vi "Actor Core.vi"(8 "error in":errorcluster, 11 "Nested in":refnum<class "Text based Communications Test.lvclass">) -> (0 "error out":errorcluster, 3 "Actor out":refnum<class "Actor.lvclass">)   [LabVIEW 2017, in "Text based Communications Test.lvlib" / "Text based Communications Test.lvclass"]
doc: "(<B>Filename</B>: Actor Framework.lvlib:Actor.lvclass:Actor Core.vi)\n\nReceives messages to the actor, reacts to them, and initiates any error handling that may shut the actor down.\n\nDescendant classes may override this VI to append parallel tasks for the actor to complete while it handles messages. Overrides use the Call Parent Method node."
uses:
  Text based Communications Test.lvclass
  C:/Program Files (x86)/National Instruments/LabVIEW 2017/vi.lib/ActorFramework/Actor/Actor.lvclass
  <vilib>/ActorFramework/Actor/Actor.lvclass
  File based Comm Helper Loop States.ctl
  <vilib>/ActorFramework/Message Enqueuer/Message Enqueuer.lvclass
  File Data Format.ctl
  Text based Communications Test.lvclass/Text based Communications Test.ctl
  <vilib>/ActorFramework/Actor/Actor.lvclass/Actor.ctl
  <vilib>/ActorFramework/Message Enqueuer/Message Enqueuer.lvclass/Message Enqueuer.ctl
  Test/Test Messages/Update Test Progress Msg/Update Test Progress Msg.lvclass/Update Test Progress Msg.ctl
  Text based Communications Test Messages/Validate Response Msg/Validate Response Msg.lvclass/Validate Response Msg.ctl
  <vilib>/ActorFramework/Message Enqueuer/Init from Existing Queue.vi
  <vilib>/ActorFramework/Message Enqueuer/Enqueue.vi
  Test/Test Messages/Update Test Progress Msg/Update Test Progress Msg.lvclass
  C:/Program Files (x86)/National Instruments/LabVIEW 2017/vi.lib/ActorFramework/Message/Message.lvclass
  Text based Communications Test Messages/Validate Response Msg/Validate Response Msg.lvclass
  <vilib>/ActorFramework/Message Priority Queue/Priority Enqueue.vi
  Test/Test/Test.lvclass
  Text based Communications Test.lvlib
panel:
  out "Table":i32[](listbox)
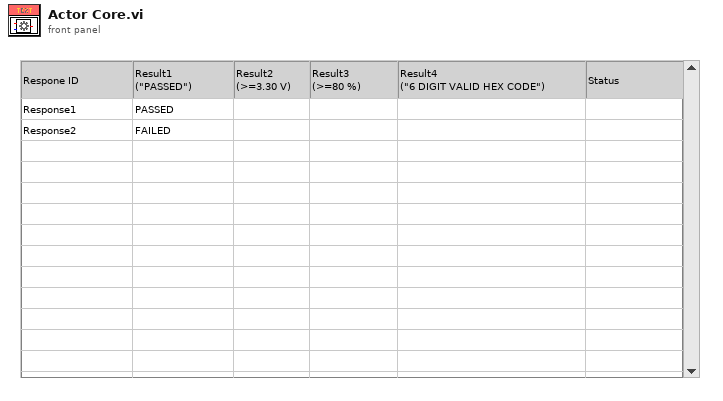
[diagram p1: front panel]
types:
  T1 = typedef "Text based Communications Test.lvlib/File Data Format.ctl" = cluster{"Response ID":string, "Value":cluster{"Result1":string, "Result2":dbl, "Result3":string, "Result4":string}}
  T2 = cluster{"Self Enqueuer":refnum<class "Message Enqueuer.lvclass">, "raw text":string, "File Type":string, "Array":T1[], "Test Name":string, "Test Configuration":cluster{"Path":path}}
  T3 = typedef "Text based Communications Test.lvlib/File based Comm Helper Loop States.ctl" = enum16{"Poll", "Init", "Read Test Case", "Read Input Text File", "Parse Data", "Validate", "Update Result", "Stream Data to Actor", "Error", "Exit"}
  T4 = typedef "Paths.ctl" = cluster{"Data Directory":path, "Test Config Dir":path, "Error Logs":path, "Event Logs":path, "Settings.Json":path, "Reports Directory":path}
  T5 = cluster{"Response ID":string, "Value":cluster{"Result1":string, "Result2":dbl, "Result3":string, "Result4":string}}[]
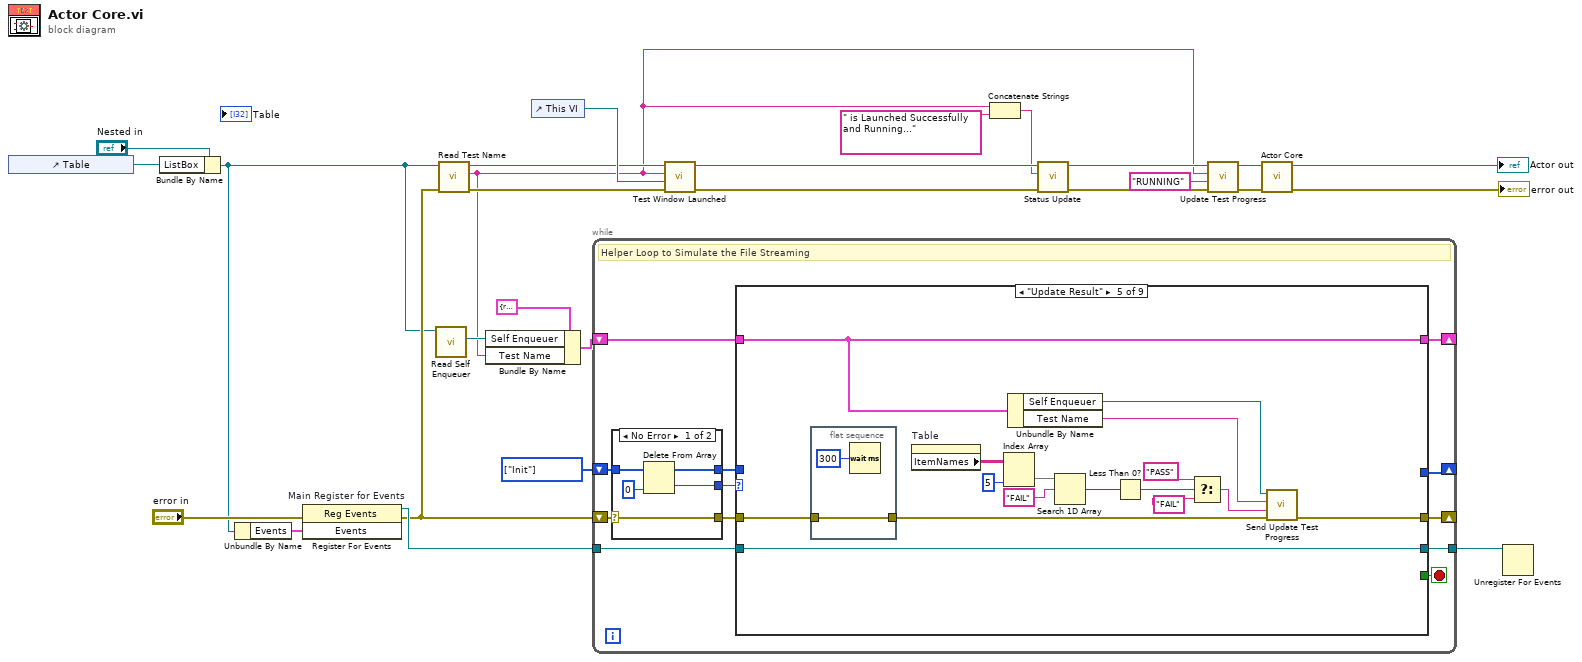
[diagram p0: block diagram]
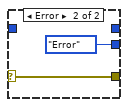
[diagram p2: hidden frame]
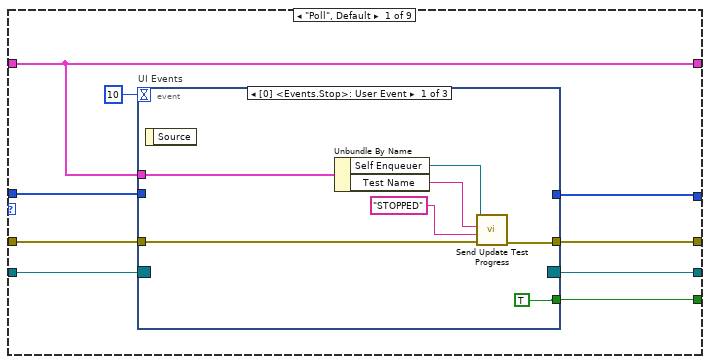
[diagram p3: hidden frame]
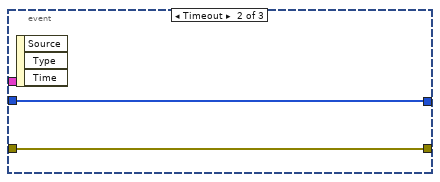
[diagram p4: hidden frame]
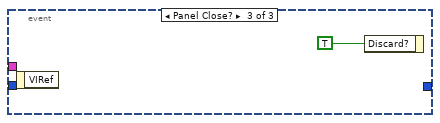
[diagram p5: hidden frame]
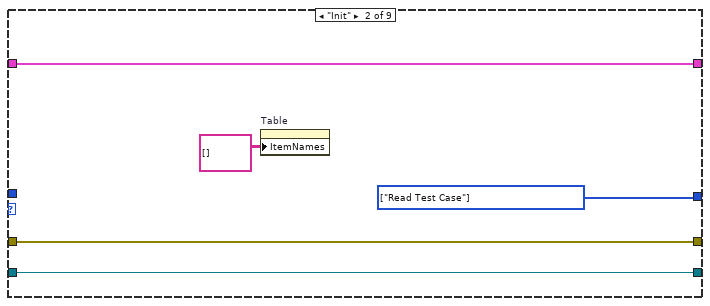
[diagram p6: hidden frame]
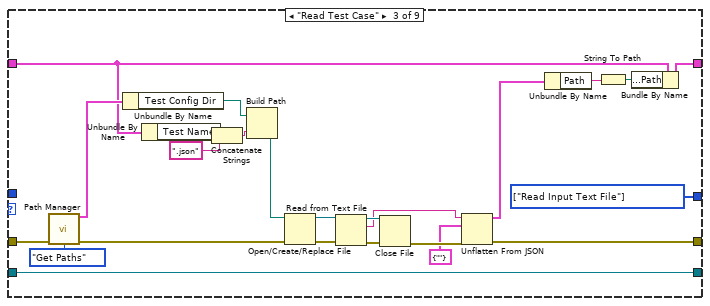
[diagram p7: hidden frame]
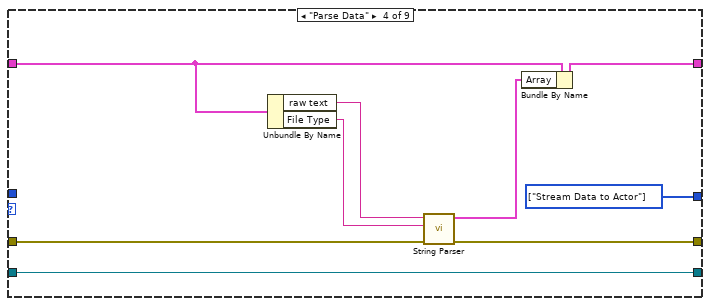
[diagram p8: hidden frame]
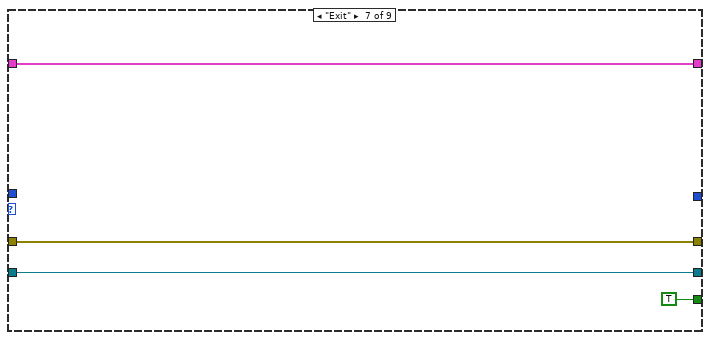
[diagram p10: hidden frame]
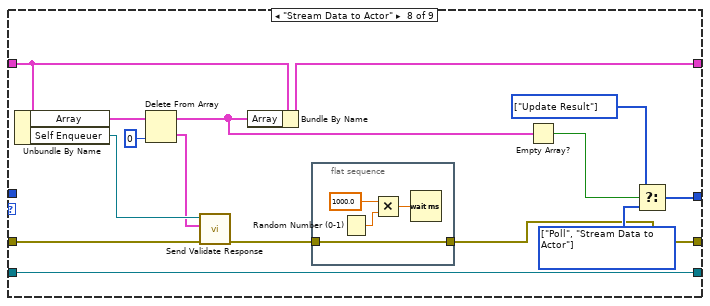
[diagram p11: hidden frame]
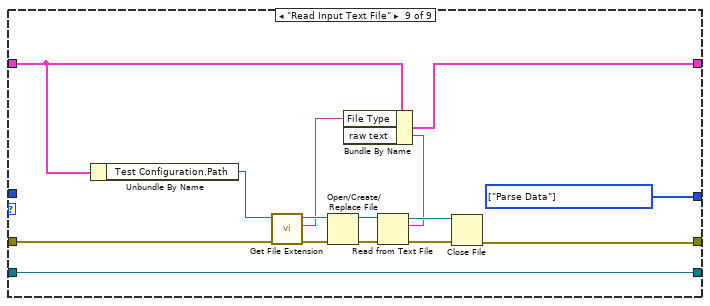
[diagram p12: hidden frame]
diagram:
  w17 = T3[] [enum."Init"] items=["Poll", "Init", "Read Test Case", "Read Input Text File", "Parse Data", "Validate", "Update Result", "Stream Data to Actor", "Error", "Exit"]
  n1 = control-ref of="Table"() -> (w2:refnum<vi>)
  n2 = Bundle By Name(cluster="Nested in", "ListBox"=w2) -> (w3:refnum<class "Text based Communications Test.lvclass">)
  n3 = Unbundle By Name(w3) -> ("Events"=w22:cluster{"Stop":refnum<user-event>})
  n4 = register-events "Main Register for Events"(error in="error in", w22) -> (reference out=w23:refnum<event-registration>, error out=w18:errorcluster)  [unwired: 1 in]
  n5 = call <vilib>:"Read Self Enqueuer.vi"("Actor"=w3) -> ("Self Enqueuer"=w4:refnum<class "Message Enqueuer.lvclass">)  [unwired: 10 in]
  n6 = call-dynamic "Read Test Name.vi"("Test in"=w3) -> ("Test Name"=w1:string, "Test out"=w10:refnum<class "Text based Communications Test.lvclass">)  [unwired: 8 in, 1 out]
  n7 = Bundle By Name(cluster=T2 {"Self Enqueuer"=refnum, "raw text"="", "File Type"="", "Array"=[], "Test Name"="", "Test Configuration"={"Path"=path ""}}, "Self Enqueuer"=w4, "Test Name"=w1) -> (w5:T2)
  n8 = control-ref of="This VI"() -> (w19:refnum<vi>)
  n9 = while {
    tunnel: w23 -> [w37]
    tunnel: [w35] -> w21
    shift-right: [w30] -> _
    shift-left: w17 -> [w31]
    shift-right: [w34] -> _
    shift-left: w18 -> [w32]
    shift-right: [w28] -> _
    shift-left: w5 -> [w29]
    stop <- w36 stop-if-true
    # "Helper Loop to Simulate the File Streaming"
    n10 = case shown="No Error" w32 {
      selector: w32 -> [w41 w44]
      tunnel: [w41 w44] -> w33
      tunnel: w31 -> [w42 _]
      tunnel: [w40 _] -> w26
      tunnel: [w38 File_based_Comm_Helper_Loop_States."Error" ("Enum")] -> w27
      frame No Error {
        n11 = Delete From Array(array=w42, index=0) -> (deleted portion=w38:T3, array with subset deleted=w40:T3[])  [unwired: 1 in]
      }
      frame Error {
      }
    }
    n12 = case shown="\"Update Result\"" w27 {
      tunnel: w37 -> [w53 w68 w92 w101 w117 w122 w124 w141 w160]
      tunnel: [w52 _ _ _ _ _ TRUE _ _] -> w36
      tunnel: [w51 w68 w92 w101 w117 w122 w124 w141 w160] -> w35
      tunnel: w33 -> [w50 w67 w91 w100 w103 w120 w126 w130 w154]
      tunnel: [w48 w67 w76 w99 w104 w120 w126 w127 w150] -> w34
      tunnel: [w46 w64 w69 w93 _ _ _ w133 w149] -> w30
      tunnel: w29 -> [w45 w66 w74 w96 w105 w121 w123 w140 w147]
      tunnel: [w45 w66 w73 w98 w105 w121 w123 w137 w148] -> w28
      tunnel: w26 -> [w47 _ _ _ _ _ _ _ _]
      frame "Poll", Default {
        n13 = event "UI Events" shown="[0] <Events.Stop>: User Event" {
          selector: w53 -> [_ _ _]
          dyn-events: [_ _ _] -> w51
          timeout: 10 -> [_ _ _]
          tunnel: [TRUE _ _] -> w52
          tunnel: w50 -> [w55 w62 _]
          tunnel: [w54 w62 _] -> w48
          tunnel: w47 -> [_ w61 _]
          tunnel: [_ w61 _] -> w46
          tunnel: w45 -> [w57 _ _]
          event User Event {
            n14 = event-data() -> ()  [unwired: 1 in, 1 out]
            n15 = Unbundle By Name(w57) -> ("Self Enqueuer"=w56:refnum<class "Message Enqueuer.lvclass">, "Test Name"=w58:string)
            n16 = call "Send Update Test Progress.vi"("error in (no error)"=w55, "State"="STOPPED", "Test Name"=w58, "Message Enqueuer"=w56) -> ("error out"=w54:errorcluster)  [unwired: 6 in, 1 out]
          }
          event Timeout {
            n17 = event-data() -> ()  [unwired: 1 in, 3 out]
          }
          event Panel Close? {
            n18 = event-data() -> ()  [unwired: 1 in, 1 out]
            n19 = event-data("Discard?"=TRUE) -> ()  [unwired: 1 in, 1 out]
          }
        }
      }
      frame "Init" {
        w64 = T3[] [enum."Read Test Case"] items=["Poll", "Init", "Read Test Case", "Read Input Text File", "Parse Data", "Validate", "Update Result", "Stream Data to Actor", "Error", "Exit"] ("t")
        n20 = property on="Table" class="MCListbox (strict)"("ItemNames"=string[][] [] ("Item Names")) -> ()  [unwired: 2 in, 2 out]
      }
      frame "Read Test Case" {
        w69 = T3[] [enum."Read Input Text File"] items=["Poll", "Init", "Read Test Case", "Read Input Text File", "Parse Data", "Validate", "Update Result", "Stream Data to Actor", "Error", "Exit"] ("t")
        n21 = call "Path Manager.vi"("Error in (no error)"=w91, "Options"=enum16{"Get Paths", "Init Paths"}."Get Paths") -> ("Cluster"=w89:T4, "Error out"=w80:errorcluster)  [unwired: 12 in]
        n22 = Unbundle By Name(w89) -> ("Test Config Dir"=w88:path)
        n23 = Unbundle By Name(w74) -> ("Test Name"=w87:string)
        n24 = Concatenate Strings(w87, ".json" ("string")) -> (w86:string)
        n25 = Build Path(base path=w88, name or relative path=w86) -> (appended path=w79:path)
        n26 = Open/Create/Replace File(file path (use dialog)=w79, error in=w80) -> (refnum out=w83:refnum<file>, error out=w84:errorcluster)  [unwired: 4 in, 1 out]
        n27 = Read from Text File(file (use dialog)=w83, error in=w84) -> (refnum out=w81:refnum<file>, text=w78:string, error out=w82:errorcluster)  [unwired: 2 in, 1 out]
        n28 = Close File(refnum=w81, error in=w82) -> (error out=w77:errorcluster)  [unwired: 1 out]
        n29 = Unflatten From JSON(JSON string=w78, type and defaults=cluster{"Path":string} {"Path"=""}, error in (no error)=w77) -> (value=w72:cluster{"Path":string}, error out=w76:errorcluster)  [unwired: 4 in]
        n30 = Unbundle By Name(w72) -> ("Path"=w71:string)
        n31 = String To Path(string=w71) -> (path=w70:path)
        n32 = Bundle By Name(cluster=w74, "Test Configuration.Path"=w70) -> (w73:T2)
      }
      frame "Parse Data" {
        w93 = T3[] [enum."Stream Data to Actor"] items=["Poll", "Init", "Read Test Case", "Read Input Text File", "Parse Data", "Validate", "Update Result", "Stream Data to Actor", "Error", "Exit"]
        n33 = Unbundle By Name(w96) -> ("raw text"=w95:string, "File Type"=w94:string)
        n34 = call "String Parser.vi"("Error in (no error)"=w100, "File Type"=w94, "raw string"=w95) -> ("Error out"=w99:errorcluster, "Array"=w97:T5)  [unwired: 7 in]
        n35 = Bundle By Name(cluster=w96, "Array"=w97) -> (w98:T2)
      }
      frame "Update Result" {
        n36 = flat-sequence {
          tunnel: w103 -> [w119]
          tunnel: [w119] -> w102
          frame #0 {
            n37 = Wait (ms)(milliseconds to wait=u32 300) -> ()  [unwired: 1 out]
          }
        }
        n38 = property on="Table" class="MCListbox (strict)"() -> ("ItemNames"=w106:string[][])  [unwired: 2 in, 2 out]
        n39 = Index Array(array=w106, index (col)=5 ("disabled index (col)")) -> (element=w113:string[])  [unwired: 1 in]
        n40 = Unbundle By Name(w105) -> ("Self Enqueuer"=w116:refnum<class "Message Enqueuer.lvclass">, "Test Name"=w115:string)
        n41 = Search 1D Array(1D array=w113, element="FAIL") -> (index of element=w111:i32)  [unwired: 1 in]
        n42 = Less Than 0?(x=w111) -> (x < 0?=w110:bool)
        n43 = Select(t="PASS" ("State"), s=w110, f="FAIL" ("State")) -> (s? t:f=w107:string)
        n44 = call "Send Update Test Progress.vi"("error in (no error)"=w102, "State"=w107, "Test Name"=w115, "Message Enqueuer"=w116) -> ("error out"=w104:errorcluster)  [unwired: 6 in, 1 out]
      }
      frame "Error" {
      }
      frame "Exit" {
      }
      frame "Stream Data to Actor" {
        w129 = T3[] [enum."Update Result"] items=["Poll", "Init", "Read Test Case", "Read Input Text File", "Parse Data", "Validate", "Update Result", "Stream Data to Actor", "Error", "Exit"] ("t")
        w134 = T3[] [enum."Poll", enum."Stream Data to Actor"] items=["Poll", "Init", "Read Test Case", "Read Input Text File", "Parse Data", "Validate", "Update Result", "Stream Data to Actor", "Error", "Exit"]
        n45 = Unbundle By Name(w140) -> ("Array"=w139:T1[], "Self Enqueuer"=w132:refnum<class "Message Enqueuer.lvclass">)
        n46 = Delete From Array(array=w139, index=0) -> (deleted portion=w131:T1, array with subset deleted=w136:T1[])  [unwired: 1 in]
        n47 = call "Send Validate Response.vi"("error in (no error)"=w130, "Response Data"=w131, "Message Enqueuer"=w132) -> ("error out"=w128:errorcluster)  [unwired: 7 in, 1 out]
        n48 = Bundle By Name(cluster=w140, "Array"=w136) -> (w137:T2)
        n49 = flat-sequence {
          tunnel: w128 -> [w145]
          tunnel: [w145] -> w127
          frame #0 {
            n50 = Random Number (0-1)() -> (number: 0 to 1=w144:dbl)
            n51 = Multiply(x=1000.0, y=w144) -> (x*y=w142:dbl)
            n52 = Wait (ms)(milliseconds to wait=w142) -> ()  [unwired: 1 out]
          }
        }
        n53 = Empty Array?(array=w136) -> (empty?=w135:bool)
        n54 = Select(t=w129, s=w135, f=w134) -> (s? t:f=w133:T3[])
      }
      frame "Read Input Text File" {
        w149 = T3[] [enum."Parse Data"] items=["Poll", "Init", "Read Test Case", "Read Input Text File", "Parse Data", "Validate", "Update Result", "Stream Data to Actor", "Error", "Exit"]
        n55 = Unbundle By Name(w147) -> ("Test Configuration.Path"=w146:path)
        n56 = call <vilib>:"Get File Extension.vi"("error in (no error)"=w154, "file"=w146) -> ("error out"=w153:errorcluster, "lowercase file extension"=w155:string, "dup file"=w156:path)  [unwired: 5 in, 2 out]
        n57 = Open/Create/Replace File(file path (use dialog)=w156, error in=w153) -> (refnum out=w159:refnum<file>, error out=w152:errorcluster)  [unwired: 4 in, 1 out]
        n58 = Read from Text File(file (use dialog)=w159, error in=w152) -> (refnum out=w158:refnum<file>, text=w157:string, error out=w151:errorcluster)  [unwired: 2 in, 1 out]
        n59 = Bundle By Name(cluster=w147, "File Type"=w155, "raw text"=w157) -> (w148:T2)
        n60 = Close File(refnum=w158, error in=w151) -> (error out=w150:errorcluster)  [unwired: 1 out]
      }
    }
  }
  n61 = call-dynamic "Test Window Launched.vi"("error in (no error)"=w18, "VI Refnum"=w19, "Window Name"=w1, "Test in"=w10) -> ("error out"=w8:errorcluster, "Test out"=w16:refnum<class "Text based Communications Test.lvclass">)  [unwired: 6 in]
  n62 = Concatenate Strings(w1, " is Launched Successfully and Running..." ("Status")) -> (w15:string)
  n63 = call-dynamic "Status Update.vi"("Status"=w15, "Test in"=w16) -> ("Test out"=w13:refnum<class "Text based Communications Test.lvclass">)  [unwired: 8 in, 1 out]
  n64 = call-dynamic "Update Test Progress.vi"("error in (no error)"=w8, "State"="RUNNING", "Test Name"=w1, "Test in"=w13) -> ("error out"=w7:errorcluster, "Test out"=w12:refnum<class "Text based Communications Test.lvclass">)  [unwired: 6 in]
  n65 = call-parent "Actor Core.vi"("error in"=w7, "Actor in"=w12) -> ("error out"=→"error out":errorcluster, "Actor out"=→"Actor out":refnum<class "Actor.lvclass">)  [unwired: 8 in]
  n66 = Unregister For Events(event registration refnum=w21) -> ()  [unwired: 1 in, 1 out]
